vi "Camera_Crop_Y_Axis.vi"(8 "Camera":T1, 10 "Detect Movement":bool, 11 "input cluster":T2={"Pinch-valve"="", "XLP 6000 Pump"="", "Camera1"="", "Camera2"="", "Img_Capt"=FALSE, "Actuator"=FALSE, "Pump"=FALSE, "Cam 1"=FALSE, "Cam 2"=FALSE, "Empty_Refill"=FALSE, "Crop"=FALSE, "Light intensity"=0, "Exposure Time"=0.0, "Sample Name"="", "Operator"="", "Calibration 1"=path "", "Calibration 2"=path "", "Framerate"=0, "Timeout Sample"=0, "Collection date"="", "Sample size threshold"=0, "Empty start"=0, "Command"="", "Station"="", "Species Name"="", "Other Notes"="", "Aperture"=enum."Item 0", "Image Process Queue Size"=0, "Image Save Queue Size"=0, "Overload threshold"=0, "Max Framerate"=0, "Rectangle 1"={"Left"=0, "Top"=0, "Right"=0, "Bottom"=0, "Rotation"=0.0}, "Rectangle 2"={"Left"=0, "Top"=0, "Right"=0, "Bottom"=0, "Rotation"=0.0}, "Detection Region %"=200.0, "Detect 1"=path "", "Detect 2"=path "", "Max large object threshold"=500, "Open(T)/Close(F)"=FALSE, "Img_Capt Begin"=FALSE, "Dispense Speed"=0, "Flush Size"=0, "Location"="", "Latitude"="", "Longitude"="", "Determiner"="", "Sex"="", "Camera1_Img"=refnum, "Camera2_Img"=refnum, "Img1_Orig_Disp"=refnum, "Img2_Orig_Disp"=refnum, "Img1_Orig_RGB"=refnum, "Img2_Orig_RGB"=refnum, "Blue_Plane_Extract"=refnum, "Subtracted_Plane"=refnum, "Img1_Binary"=refnum, "Img2_Binary"=refnum, "Crop_Mask"=refnum, "Img1_Save"=refnum, "Img2_Save"=refnum, "Img1_Cali_Full"=refnum, "Img2_Cali_Full"=refnum, "Img1_Cali_Detect"=refnum, "Img2_Cali_Detect"=refnum, "Cam 1 queue"=refnum, "Cam 2 queue"=refnum, "Cam 1 - save queue"=refnum, "Cam 2 - save queue"=refnum, "Overlay_Ring"=0, "SystemVersion"=0, "System Serial"="", "Legacy Cam Attributes"=FALSE, "Camera Orientation 1"="", "Camera Orientation 2"="", "Pixel to mm 1"=0.0, "Pixel to mm 2"=0.0, "CAM1 Model"=enum."a2A5328-15ucBAS", "CAM2 Model"=enum."a2A5328-15ucBAS", "Flush Insect"=FALSE, "Pump Size"=FALSE, "Barcode"="", "Phase3"=FALSE, "Mega F3"="", "Container nr."=0.0, "Flush Error"=TRUE, "Start System"=FALSE, "Size Interval"=0.0, "Mun. of containers"=0.0, "Sorting sys."=FALSE, "Initial size"=0.0} {"SystemVersion" items=["Standard", "XL"]; "Overlay_Ring" items=["Session Data", "Extended Setup", "Buffer", "Camera", "Dispenser", "Stats", "Connections"]; "Flush Size" min=1; "Dispense Speed" min=1; "Rectangle 2"."Rotation" format="%.2f"; "Rectangle 2"."Left" scale=0.0..1024.0; "Rectangle 2"."Right" scale=0.0..1024.0; "Rectangle 1"."Rotation" format="%.2f"; "Rectangle 1"."Left" scale=0.0..1024.0; "Rectangle 1"."Right" scale=0.0..1024.0; "Max Framerate" min=1; "Overload threshold" min=1; "Image Save Queue Size" min=1; "Image Process Queue Size" min=1; "Empty start" min=1; "Sample size threshold" min=1; "Framerate" min=1; "Light intensity" scale=0.0..100.0}) -> (1 "Height":i64, 3 "OffsetY":i64)   [LabVIEW 2024]
uses:
  controls/Data.ctl
  <vilib>/userDefined/High Color/IMAQdx.ctl
  <vilib>/vision/Image Controls.llb/IMAQ Image.ctl
  Camera_ID.ctl
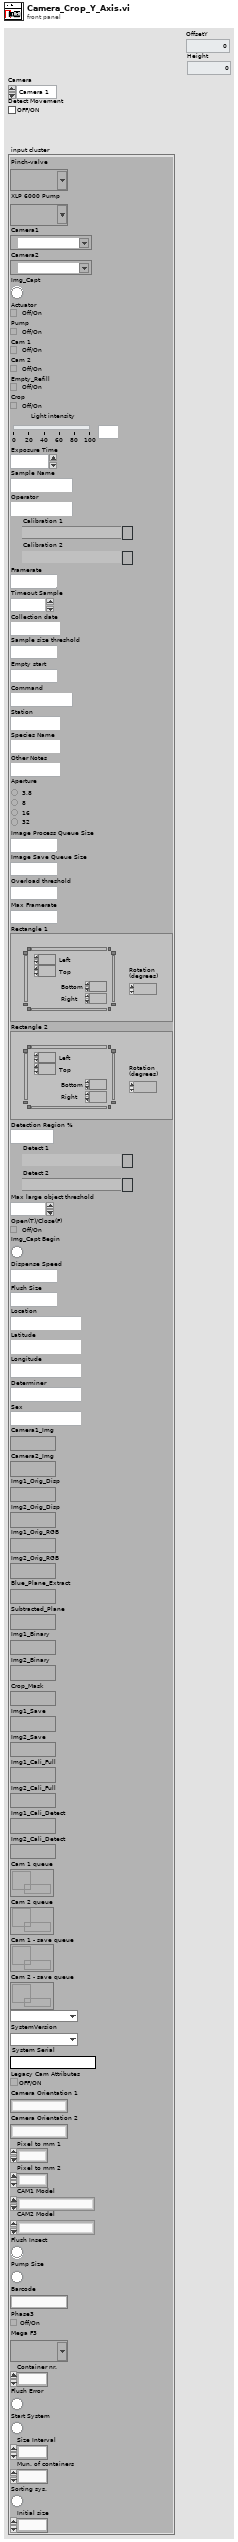
[diagram p1: front panel]
types:
  T1 = typedef "Camera_ID.ctl" = enum16{"Camera 1", "Camera 2"}
  T2 = typedef "Data.ctl" = cluster{"Pinch-valve":refnum<visa-resource-name>, "XLP 6000 Pump":refnum<visa-resource-name>, "Camera1":T3, "Camera2":T3, "Img_Capt":bool, "Actuator":bool, "Pump":bool, "Cam 1":bool, "Cam 2":bool, "Empty_Refill":bool, "Crop":bool, "Light intensity":i32, "Exposure Time":dbl, "Sample Name":string, "Operator":string, "Calibration 1":path, "Calibration 2":path, "Framerate":i32, "Timeout Sample":i32, "Collection date":string, "Sample size threshold":i32, "Empty start":u32, "Command":string, "Station":string, "Species Name":string, "Other Notes":string, "Aperture":enum32{"Item 0", "Item 1", "Item 2", "Item 3"}, "Image Process Queue Size":i32, "Image Save Queue Size":i32, "Overload threshold":i32, "Max Framerate":i32, "Rectangle 1":T4, "Rectangle 2":T4, "Detection Region %":dbl, "Detect 1":path, "Detect 2":path, "Max large object threshold":i32, "Open(T)/Close(F)":bool, "Img_Capt Begin":bool, "Dispense Speed":i32, "Flush Size":i32, "Location":string, "Latitude":string, "Longitude":string, "Determiner":string, "Sex":string, "Camera1_Img":T5, "Camera2_Img":T5, "Img1_Orig_Disp":T5, "Img2_Orig_Disp":T5, "Img1_Orig_RGB":T5, "Img2_Orig_RGB":T5, "Blue_Plane_Extract":T5, "Subtracted_Plane":T5, "Img1_Binary":T5, "Img2_Binary":T5, "Crop_Mask":T5, "Img1_Save":T5, "Img2_Save":T5, "Img1_Cali_Full":T5, "Img2_Cali_Full":T5, "Img1_Cali_Detect":T5, "Img2_Cali_Detect":T5, "Cam 1 queue":refnum<queue>, "Cam 2 queue":refnum<queue>, "Cam 1 - save queue":refnum<queue>, "Cam 2 - save queue":refnum<queue>, "Overlay_Ring":u16, "SystemVersion":u16, "System Serial":string, "Legacy Cam Attributes":bool, "Camera Orientation 1":string, "Camera Orientation 2":string, "Pixel to mm 1":dbl, "Pixel to mm 2":dbl, "CAM1 Model":enum16{"a2A5328-15ucBAS", "acA1920-155uc"}, "CAM2 Model":enum16{"a2A5328-15ucBAS", "acA1920-155uc"}, "Flush Insect":bool, "Pump Size":bool, "Barcode":string, "Phase3":bool, "Mega F3":refnum<visa-resource-name>, "Container nr.":dbl, "Flush Error":bool, "Start System":bool, "Size Interval":dbl, "Mun. of containers":dbl, "Sorting sys.":bool, "Initial size":dbl}
  T3 = typedef "IMAQdx.ctl" = refnum<k21>
  T4 = typedef "IMAQ Rectangle" = cluster{"Left":i32, "Top":i32, "Right":i32, "Bottom":i32, "Rotation":dbl}
  T5 = typedef "IMAQ Image.ctl" = refnum<image>
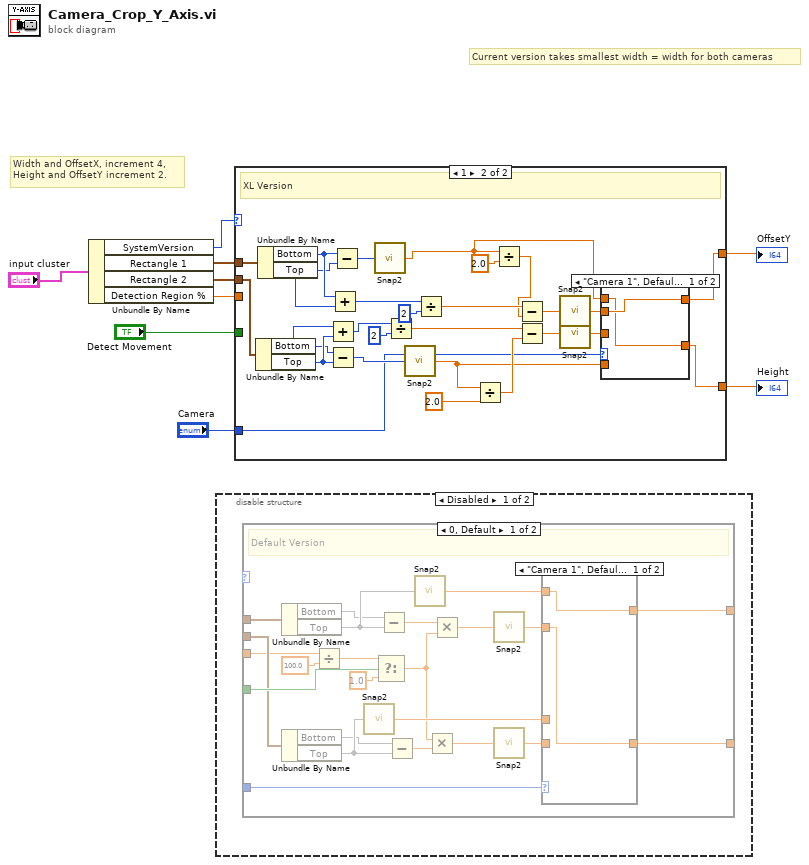
[diagram p0: block diagram]
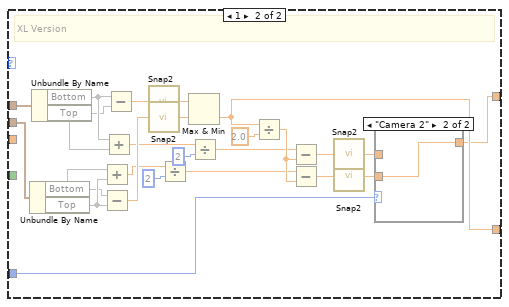
[diagram p3: hidden frame]
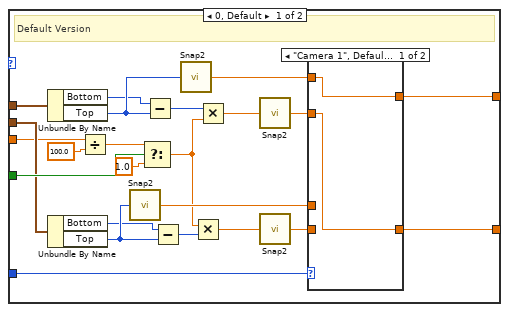
[diagram p6: hidden frame]
diagram:
  # "Current version takes smallest width = width for both cameras"
  # "Width and OffsetX, increment 4,\nHeight and OffsetY increment 2."
  n1 = Unbundle By Name("input cluster") -> ("SystemVersion"=w1:u16, "Rectangle 1"=w6:T4, "Rectangle 2"=w7:T4, "Detection Region %"=w4:dbl)
  n2 = disable-structure shown="Disabled" {
    frame Disabled {
      n3 = case shown="0, Default" {
        selector: _ -> [_ _]
        tunnel: _ -> [w27 _]
        tunnel: _ -> [w26 w42]
        tunnel: _ -> [w25 w41]
        tunnel: _ -> [w24 w43]
        tunnel: _ -> [w19 _]
        tunnel: [w18 w45] -> _
        tunnel: [w17 w44] -> _
        frame 0, Default {
          # "Default Version"
          n4 = Unbundle By Name(w25) -> ("Bottom"=w14, "Top"=w16)
          n5 = Unbundle By Name(w26) -> ("Bottom"=w13, "Top"=w15)
          n6 = Divide(x=w19, y=100.0 ("x")) -> (x/y=w29:dbl)
          n7 = call "Snap2.vi"("x"=w15) -> ("x out"=w23:dbl)
          n8 = Select(t=w29, s=w27, f=1.0 ("t")) -> (s? t:f=w10:dbl)
          n9 = Subtract(x=w14, y=w16) -> (x-y=w31:dbl)
          n10 = Subtract(x=w13, y=w15) -> (x-y=w32:dbl)
          n11 = call "Snap2.vi"("x"=w16) -> ("x out"=w21:dbl)
          n12 = Multiply(x=w10, y=w32) -> (x*y=w11:dbl)
          n13 = Multiply(x=w31, y=w10) -> (x*y=w12:dbl)
          n14 = call "Snap2.vi"("x"=w12) -> ("x out"=w20:dbl)
          n15 = call "Snap2.vi"("x"=w11) -> ("x out"=w22:dbl)
          n16 = case shown="\"Camera 1\", Default" w24 {
            tunnel: w23 -> [_ w36]
            tunnel: [w34 w36] -> w17
            tunnel: w20 -> [w33 _]
            tunnel: [w33 w35] -> w18
            tunnel: w21 -> [w34 _]
            tunnel: w22 -> [_ w35]
            frame "Camera 1", Default {
            }
            frame "Camera 2" {
            }
          }
        }
        frame 1 {
          # "XL Version"
          n17 = Unbundle By Name(w42) -> ("Bottom"=w37, "Top"=w38)
          n18 = Unbundle By Name(w41) -> ("Bottom"=w40, "Top"=w39)
          n19 = Add(x=w37, y=w38) -> (x+y=w52:dbl)
          n20 = Subtract(x=w37, y=w38) -> (x-y=w59:dbl)
          n21 = Add(x=w40, y=w39) -> (x+y=w49:dbl)
          n22 = Subtract(x=w40, y=w39) -> (x-y=w56:dbl)
          n23 = call "Snap2.vi"("x"=w56) -> ("x out"=w57:dbl)
          n24 = call "Snap2.vi"("x"=w59) -> ("x out"=w60:dbl)
          n25 = Divide(x=w52, y=2) -> (x/y=w54:dbl)
          n26 = Max & Min(x=w57, y=w60) -> (min(x,y)=w45:dbl)  [unwired: 1 out]
          n27 = Divide(x=w49, y=2) -> (x/y=w51:dbl)
          n28 = Divide(x=w45, y=2.0) -> (x/y=w55:dbl)
          n29 = Subtract(x=w51, y=w55) -> (x-y=w58:dbl)
          n30 = Subtract(x=w54, y=w55) -> (x-y=w61:dbl)
          n31 = call "Snap2.vi"("x"=w58) -> ("x out"=w47:dbl)
          n32 = call "Snap2.vi"("x"=w61) -> ("x out"=w46:dbl)
          n33 = case shown="\"Camera 2\"" w43 {
            tunnel: w47 -> [w62 _]
            tunnel: [w62 w63] -> w44
            tunnel: w46 -> [_ w63]
            frame "Camera 1", Default {
            }
            frame "Camera 2" {
            }
          }
        }
      }
    }
    frame Enabled {
    }
  }
  n34 = case shown="1" w1 {
    tunnel: "Detect Movement" -> [w81 _]
    tunnel: w7 -> [w80 w101]
    tunnel: w6 -> [w79 w100]
    tunnel: "Camera" -> [w78 w102]
    tunnel: w4 -> [w73 _]
    tunnel: [w72 w95] -> w3
    tunnel: [w71 w103] -> w2
    frame 0, Default {
      # "Default Version"
      n35 = Unbundle By Name(w79) -> ("Bottom"=w68:i32, "Top"=w70:i32)
      n36 = Unbundle By Name(w80) -> ("Bottom"=w67:i32, "Top"=w69:i32)
      n37 = Divide(x=w73, y=100.0 ("x")) -> (x/y=w83:dbl)
      n38 = call "Snap2.vi"("x"=w69) -> ("x out"=w77:dbl)
      n39 = Select(t=w83, s=w81, f=1.0 ("t")) -> (s? t:f=w64:dbl)
      n40 = Subtract(x=w68, y=w70) -> (x-y=w85:i32)
      n41 = Subtract(x=w67, y=w69) -> (x-y=w86:i32)
      n42 = call "Snap2.vi"("x"=w70) -> ("x out"=w75:dbl)
      n43 = Multiply(x=w64, y=w86) -> (x*y=w65:dbl)
      n44 = Multiply(x=w85, y=w64) -> (x*y=w66:dbl)
      n45 = call "Snap2.vi"("x"=w66) -> ("x out"=w74:dbl)
      n46 = call "Snap2.vi"("x"=w65) -> ("x out"=w76:dbl)
      n47 = case shown="\"Camera 1\", Default" w78 {
        tunnel: w77 -> [_ w90]
        tunnel: [w88 w90] -> w71
        tunnel: w74 -> [w87 _]
        tunnel: [w87 w89] -> w72
        tunnel: w75 -> [w88 _]
        tunnel: w76 -> [_ w89]
        frame "Camera 1", Default {
        }
        frame "Camera 2" {
        }
      }
    }
    frame 1 {
      # "XL Version"
      n48 = Unbundle By Name(w101) -> ("Bottom"=w96:i32, "Top"=w97:i32)
      n49 = Unbundle By Name(w100) -> ("Bottom"=w99:i32, "Top"=w98:i32)
      n50 = Add(x=w96, y=w97) -> (x+y=w110:i32)
      n51 = Subtract(x=w96, y=w97) -> (x-y=w116:i32)
      n52 = Add(x=w99, y=w98) -> (x+y=w107:i32)
      n53 = Subtract(x=w99, y=w98) -> (x-y=w114:i32)
      n54 = call "Snap2.vi"("x"=w114) -> ("x out"=w91:dbl)
      n55 = Divide(x=w110, y=2) -> (x/y=w112:dbl)
      n56 = call "Snap2.vi"("x"=w116) -> ("x out"=w94:dbl)
      n57 = Divide(x=w107, y=2) -> (x/y=w109:dbl)
      n58 = Divide(x=w94, y=2.0) -> (x/y=w113:dbl)
      n59 = Divide(x=w91, y=2.0) -> (x/y=w92:dbl)
      n60 = Subtract(x=w109, y=w92) -> (x-y=w115:dbl)
      n61 = Subtract(x=w112, y=w113) -> (x-y=w117:dbl)
      n62 = call "Snap2.vi"("x"=w115) -> ("x out"=w105:dbl)
      n63 = call "Snap2.vi"("x"=w117) -> ("x out"=w104:dbl)
      n64 = case shown="\"Camera 1\", Default" w102 {
        tunnel: w105 -> [w119 _]
        tunnel: [w119 w121] -> w103
        tunnel: w104 -> [_ w121]
        tunnel: [w118 w120] -> w95
        tunnel: w94 -> [_ w120]
        tunnel: w91 -> [w118 _]
        frame "Camera 1", Default {
        }
        frame "Camera 2" {
        }
      }
    }
  }
  "OffsetY" <- w2
  "Height" <- w3
